vi "Constructor.vi"(8 "error in (no error)":errorcluster, 10 "PictRef":refnum<vi>, 11 "Menu in":refnum<class "Menu.lvclass">) -> (0 "error out":errorcluster, 2 "MenuSelectionEvent":refnum<user-event>, 3 "Menu out":refnum<class "Menu.lvclass">)   [LabVIEW 2021, in "Menu.lvlib" / "Menu.lvclass"]
uses:
  Menu.lvclass
  MenuSelection.ctl
  Menu.lvclass/Menu.ctl
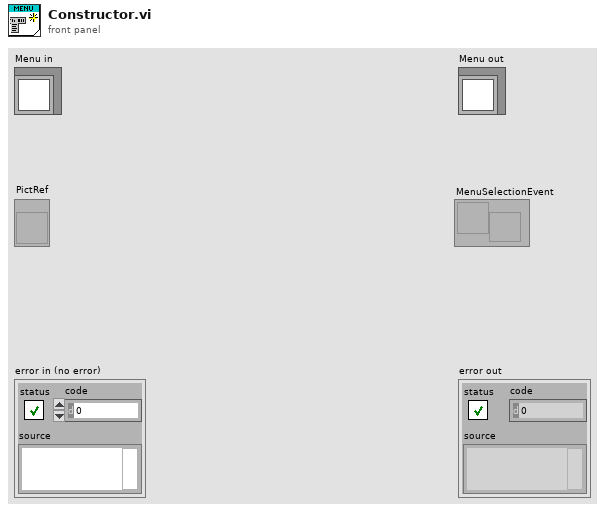
[diagram p1: front panel]
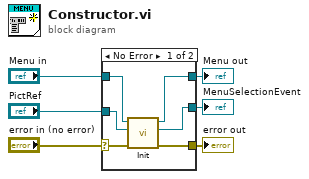
[diagram p0: block diagram]
diagram:
  n1 = case shown="No Error" "error in (no error)" {
    selector: "error in (no error)" -> [w11 w14]
    tunnel: [w9 w14] -> w5
    tunnel: [w10 w13] -> w3
    tunnel: "Menu in" -> [w12 w13]
    tunnel: "PictRef" -> [w8 _]
    tunnel: [w7 _] -> w1
    frame No Error {
      n2 = call "Init.vi"("error in (no error)"=w11, "PictRef"=w8, "Menu in"=w12) -> ("error out"=w9:errorcluster, "MenuSelectionEvent"=w7:refnum<user-event>, "Menu out"=w10:refnum<class "Menu.lvclass">)  [unwired: 6 in]
    }
    frame Error {
    }
  }
  "error out" <- w5
  "Menu out" <- w3
  "MenuSelectionEvent" <- w1
